vi "VHDI-savingStatus.vi"(8 "error in (no error)":errorcluster, 10 "data saving info":T1={"data points left"=1, "Saving?"=FALSE, "Folder Path"=path "", "filename"=""}, 11 "VG-VNA_GUI in":refnum<class "VG-VNA_GUI.lvclass">) -> (0 "error out":errorcluster, 3 "VG-VNA_GUI out":refnum<class "VG-VNA_GUI.lvclass">)   [LabVIEW 2020, in "VG-VNA_GUI.lvlib" / "VG-VNA_GUI.lvclass"]
uses:
  VG-VNA_GUI.lvclass
  data_handler/VDH-VNA_data_handler/VDH-VNA_data_handler/VDH-data_saving_info.ctl
  VG-VNA_GUI.lvclass/VG-VNA_GUI.ctl
  data_handler/VDH-VNA_data_handler/VDH-VNA_data_handler/VDH-VNA_data_handler.lvclass
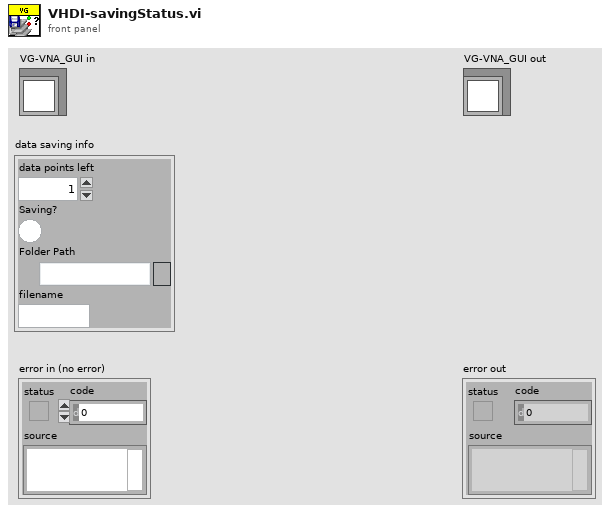
[diagram p1: front panel]
types:
  T1 = typedef "VDH-VNA_data_handler.lvlib/VDH-VNA_data_handler.lvclass/VDH-data_saving_info.ctl" = cluster{"data points left":u8, "Saving?":bool, "Folder Path":path, "filename":string}
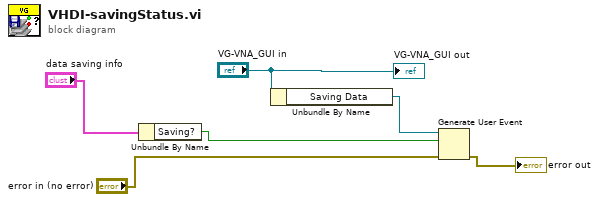
[diagram p0: block diagram]
diagram:
  n1 = Unbundle By Name("data saving info") -> ("Saving?"=w3:bool)
  n2 = Unbundle By Name("VG-VNA_GUI in") -> ("Saving Data"=w5:refnum<user-event>)
  n3 = Generate User Event(user event=w5, event data cluster=w3, error in="error in (no error)") -> (error out=→"error out":errorcluster)  [unwired: 1 in, 1 out]
  "VG-VNA_GUI out" <- "VG-VNA_GUI in"
